vi "SetPower.vi"(0 "class data in":refnum<class "MB_ENGINE.lvclass">, 7 "On":bool, 11 "error in (no error)":errorcluster) -> (4 "class data out":refnum<class "MB_ENGINE.lvclass">, 15 "error out":errorcluster)   [LabVIEW 2019, in "MB_ENGINE.lvclass"]
uses:
  MB_ENGINE.lvclass
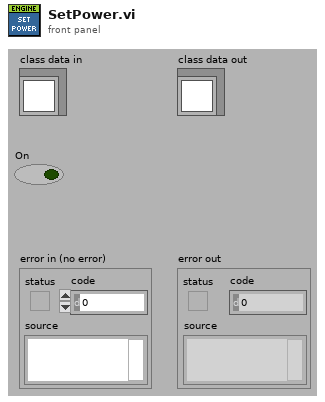
[diagram p1: front panel]
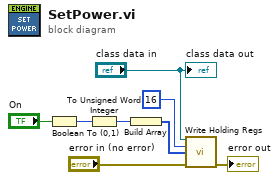
[diagram p0: block diagram]
diagram:
  n1 = Boolean To (0,1)(Boolean="On") -> (0, 1=w4:i16)
  n2 = To Unsigned Word Integer(number=w4) -> (unsigned 16bit integer=w2:u16)
  n3 = Build Array(w2) -> (w1:u16[])
  n4 = call-dynamic "Write Holding Regs.vi"("reference in"="class data in", "starting address"=u16 16, "Regs"=w1, "error in (no error)"="error in (no error)") -> ("error out"=→"error out":errorcluster)  [unwired: 11 in]
  "class data out" <- "class data in"
